vi "Add Remove Invalid Count Channel.vi"(8 "error in (no error)":errorcluster, 10 "Invalid Count Channel GUID":string, 11 "Channel Ref in":T1 format="%.0x") -> (0 "error out":errorcluster, 3 "Channel Ref out":T1 format="%.0x")   [LabVIEW 2019, in "Protection and Counter Support System Explorer.lvlib"]
uses:
  <vilib>/NI VeriStand/Custom Device API/Custom Device Item Ref.ctl
  <vilib>/NI VeriStand/Custom Device API/Custom Device Channel.ctl
  <vilib>/NI VeriStand/Custom Device API/Custom Device Channel Type.ctl
  Shared/SubVIs/Properties Lookup.vi
  Protection and Counter Support System Explorer.lvlib
  <vilib>/NI VeriStand/Custom Device API/Custom Device API.lvlib
  Shared/Protection and Counter Support Shared.lvlib
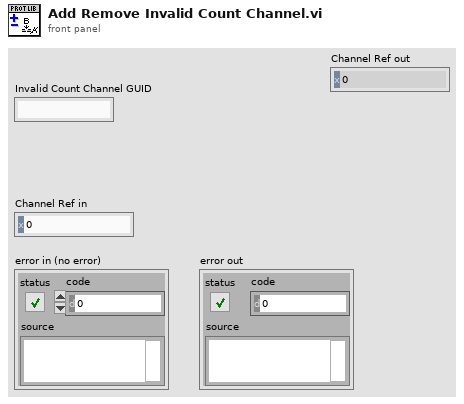
[diagram p1: front panel]
types:
  T1 = typedef "Custom Device API.lvlib/Custom Device Item Ref.ctl" = u64
  T2 = typedef "Custom Device API.lvlib/Custom Device Channel.ctl" = cluster{"Type":T3, "Units":string, "Default Value":dbl, "Faultable":bool, "Scalable":bool}
  T3 = typedef "Custom Device API.lvlib/Custom Device Channel Type.ctl" = enum16{"Input", "Output"}
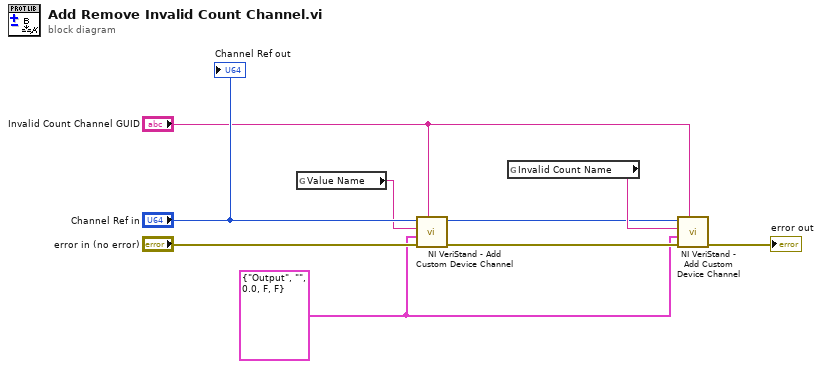
[diagram p0: block diagram]
diagram:
  w3 = T2 {"Type"=enum."Output", "Units"="", "Default Value"=0.0, "Faultable"=FALSE, "Scalable"=FALSE} ("Channel")
  n1 = global read "Properties Lookup.vi" "Value Name"() -> (w2:string)
  n2 = call <vilib>:"NI VeriStand - Add Custom Device Channel.vi"("GUID (Default Channel)"="Invalid Count Channel GUID", "error in (no error)"="error in (no error)", "Channel"=w3, "Channel Name"=w2, "Parent Ref in"="Channel Ref in") -> ("error out"=w4:errorcluster, "Parent Ref out"=w6:T1)  [unwired: 3 in, 2 out]
  n3 = global read "Properties Lookup.vi" "Invalid Count Name"() -> (w9:string)
  n4 = call <vilib>:"NI VeriStand - Add Custom Device Channel.vi"("GUID (Default Channel)"="Invalid Count Channel GUID", "error in (no error)"=w4, "Channel"=w3, "Channel Name"=w9, "Parent Ref in"=w6) -> ("error out"=→"error out":errorcluster)  [unwired: 3 in, 3 out]
  "Channel Ref out" <- "Channel Ref in"
